vi "GetRegisterIndex.vi"(0 "Data":T1, 1 "Bitfield":string, 5 "error in (no error)":errorcluster) -> (14 "Find?":bool, 15 "Empty?":bool, 16 "Index":i32, 19 "error out":errorcluster)   [LabVIEW 2017]
uses:
  Ctrl/Bitfield.ctl
  Ctrl/Register.ctl
  Ctrl/Property.ctl
  Ctrl/PhysicalChannel.ctl
  Ctrl/ScaleType.ctl
  Ctrl/Scale.ctl
  Ctrl/EnumValue.ctl
  Ctrl/Enum.ctl
  Ctrl/Caps.ctl
  Ctrl/Data.ctl
panel:
  out "Register":T5
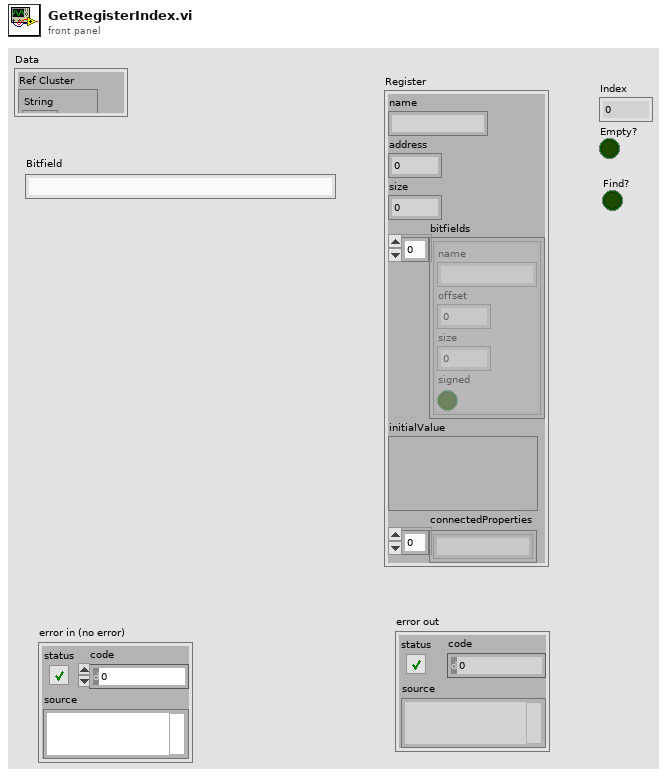
[diagram p1: front panel]
types:
  T1 = typedef "Data.ctl" = cluster{"Ref Cluster":cluster{"String":refnum<vi>, "U8":refnum<vi>, "I8":refnum<vi>, "U32":refnum<vi>, "I32":refnum<vi>, "U64":refnum<vi>, "I64":refnum<vi>, "Ring":refnum<vi>, "DBL":refnum<vi>, "Add":refnum<vi>, "Remove":refnum<vi>, "Property tree":refnum<vi>, "confirm":refnum<vi>}, "JSON Text":string, "Original JSON Text":string, "Caps":T2, "SLSC Output Tree":cluster{"Left Cell String":string, "Child Text":string[], "Child Tag":string, "Item Indent":i32, "Child Only?":bool, "Glyph Index":i32, "offline value":variant}[], "Ref Index and Control Type":cluster{"index":i32, "Datatype":string}, "Selected Type and name":cluster{"Selected Type":enum16{"Property", "Physical Channel", "Other"}, "Selected Property Name":string}, "Update whole Tree?":bool}
  T2 = typedef "Caps.ctl" = cluster{"properties":T3[], "physical channels":T4[], "registers":T5[], "scales":T7[], "enums":T9[], "productName":string}
  T3 = typedef "Property.ctl" = cluster{"name":string, "bitfield":string, "value":variant, "dataType":string, "min":variant, "max":variant, "scale":string, "access":string}
  T4 = typedef "PhysicalChannel.ctl" = cluster{"name":string, "properties":T3[]}
  T5 = typedef "Register.ctl" = cluster{"name":string, "address":i32, "size":i32, "bitfields":T6[], "initialValue":variant, "connectedProperties":string[]}
  T6 = typedef "Bitfield.ctl" = cluster{"name":string, "offset":i32, "size":i32, "signed":bool}
  T7 = typedef "Scale.ctl" = cluster{"name":string, "type":T8, "params":variant}
  T8 = typedef "ScaleType.ctl" = enum16{"NoScale", "Table", "Polynomial", "Linear"}
  T9 = typedef "Enum.ctl" = cluster{"name":string, "values":T10[]}
  T10 = typedef "EnumValue.ctl" = cluster{"name":string, "value":i32}
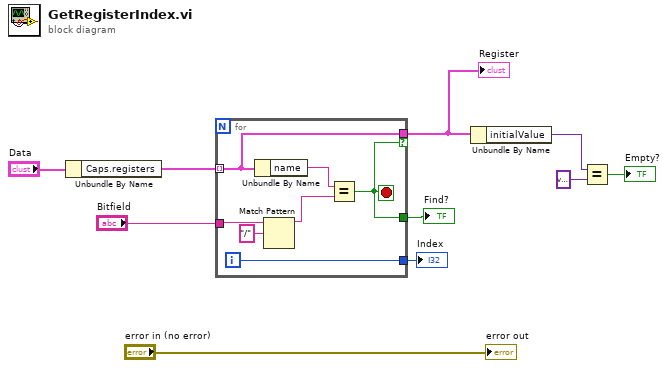
[diagram p0: block diagram]
diagram:
  n1 = Unbundle By Name("Data") -> ("Caps.registers"=w9:T5[])
  n2 = for {
    tunnel: w9 -> [w12] mode=indexing
    tunnel: "Bitfield" -> [w17]
    tunnel: [w13] -> w6
    tunnel: [w11] -> w7
    tunnel: [w12] -> w5 if=w11
    i -> [w13]
    stop <- w11 stop-if-true
    n3 = Unbundle By Name(w12) -> ("name"=w14:string)
    n4 = Match Pattern(string=w17, regular expression="/") -> (before substring=w15:string)  [unwired: 1 in, 3 out]
    n5 = Equal?(x=w14, y=w15) -> (x = y?=w11:bool)
  }
  "Find?" <- w7
  "Register" <- w5
  "Index" <- w6
  n6 = Unbundle By Name(w5) -> ("initialValue"=w4:variant)
  n7 = Equal?(x=w4, y=variant) -> (x = y?=→"Empty?":bool)
  "error out" <- "error in (no error)"
